vi "Convert String Type.vi"(5 "src byte order":T1(ring), 7 "dst byte order":T1(ring), 8 "error in (no error)":errorcluster, 9 "conversions":T2[](array[typedef]) {"converted descriptor"."buffer offset" format="%d bytes"; "unconverted descriptor"."buffer offset" format="%d bytes"}, 10 "dst buffer in":string, 11 "src buffer in":string) -> (0 "error out":errorcluster, 2 "dst buffer out":string, 3 "src buffer out":string)   [LabVIEW 2017, in "DSF Core.lvlib" / "Buffer Converter.lvclass"]
uses:
  Buffer Converter.lvclass
  Type Conversion.ctl
  Channel Descriptor.ctl
  DSF Configuration API/Public/Controls/DSF Data Type.ctl
  Shared/VIs/Sizeof 1D.vi
  Shared/VIs/Sizeof.vi
  DSF Core.lvlib
  Buffer/Buffer.lvclass
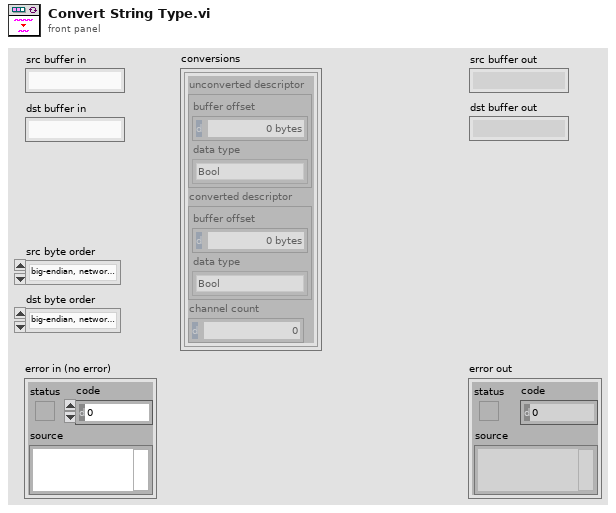
[diagram p1: front panel]
types:
  T1 = enum16{"big-endian, network order", "native, host order", "little-endian"}
  T2 = typedef "DSF Core.lvlib/Buffer Converter.lvclass/Type Conversion.ctl" = cluster{"unconverted descriptor":T3, "converted descriptor":T3, "channel count":u64}
  T3 = typedef "DSF Core.lvlib/Buffer.lvclass/Channel Descriptor.ctl" = cluster{"buffer offset":u64, "data type":T4}
  T4 = typedef "DSF Core.lvlib/DSF Data Type.ctl" = enum8{"Bool", "SGL", "DBL", "I8", "I16", "I32", "I64", "U8", "U16", "U32", "U64"}
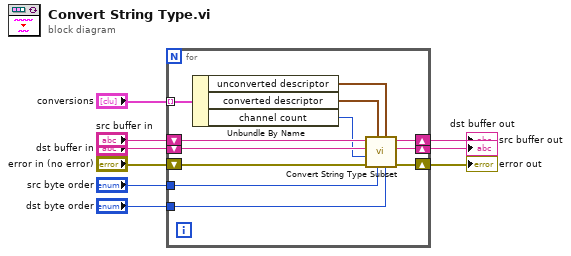
[diagram p0: block diagram]
diagram:
  n1 = for {
    shift-right: [w16] -> w3
    shift-left: "error in (no error)" -> [w21]
    shift-right: [w17] -> w4
    shift-left: "dst buffer in" -> [w20]
    shift-right: [w19] -> w2
    shift-left: "src buffer in" -> [w18]
    tunnel: "src byte order" -> [w15]
    tunnel: "dst byte order" -> [w14]
    tunnel: "conversions" -> [w13] mode=indexing
    n2 = Unbundle By Name(w13) -> ("unconverted descriptor"=w11:T3, "converted descriptor"=w12:T3, "channel count"=w10:u64)
    n3 = call "Convert String Type Subset.vi"("dst byte order"=w14, "src channel descriptor"=w11, "src byte order"=w15, "dst channel descriptor"=w12, "error in (no error)"=w21, "channel count"=w10, "dst buffer in"=w20, "src buffer in"=w18) -> ("error out"=w16:errorcluster, "dst buffer out"=w17:string, "src buffer out"=w19:string)  [unwired: 1 in]
  }
  "error out" <- w3
  "dst buffer out" <- w4
  "src buffer out" <- w2
